vi "Select Channels and Update Properties.vi"(8 "error in (no error)":errorcluster, 11 "Node Ptr":u64) -> (0 "error out":errorcluster)   [LabVIEW 2015, in "J1939 Addon System Explorer.lvlib"]
uses:
  J1939 Addon System Explorer.lvlib
  <vilib>/NI VeriStand/Custom Device Tools/Custom Device Utility Library/Custom Device Utility Library.lvlib
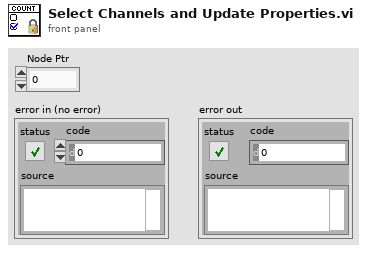
[diagram p1: front panel]
types:
  T1 = typedef "J1939 Addon System Explorer.lvlib/Protection Signal Settings.ctl" = cluster{"Input Channels":T2[], "Protection Type":T4}
  T2 = typedef "J1939 Addon System Explorer.lvlib/Protection Signal Linked Channels.ctl" = cluster{"Node Ref":T3}
  T3 = typedef "Custom Device API.lvlib/Custom Device Item Ref.ctl" = u64
  T4 = typedef "J1939 Addon Shared.lvlib/Protection Type.ctl" = enum16{"Arb ID + Bytes Checksum with Inversion", "Arb ID + Bytes CRC with Inversion", "Reversed Raw Signal Checksum with Inversion"}
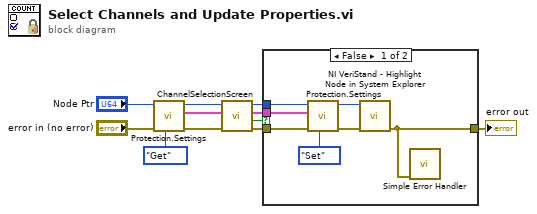
[diagram p0: block diagram]
diagram:
  n1 = call "Protection.Settings.vi"("Action"=enum8{"Get", "Set"}."Get", "error in"="error in (no error)", "Parent Ref"="Node Ptr") -> ("error out"=w3:errorcluster, "Selected Channels"=w10:T1, "Parent Ref Out"=w2:T3)  [unwired: 6 in]
  n2 = call "ChannelSelectionScreen.vi"("error in"=w3, "Selected Channels"=w10, "Parent Ref"=w2) -> ("error out"=w5:errorcluster, "Cancelled?"=w7:bool, "Selected Channels"=w11:T1, "Parent Ref Out"=w6:T3)  [unwired: 5 in]
  n3 = case shown="False" w7 {
    tunnel: w5 -> [w15 w19]
    tunnel: w6 -> [w13 _]
    tunnel: w11 -> [w14 _]
    tunnel: [w16 w19] -> w9
    frame False {
      n4 = call "Protection.Settings.vi"("Action"=enum8{"Get", "Set"}."Set", "error in"=w15, "Selected Channels"=w14, "Parent Ref"=w13) -> ("error out"=w17:errorcluster, "Parent Ref Out"=w18:T3)  [unwired: 5 in, 1 out]
      n5 = call <vilib>:"NI VeriStand - Highlight Node in System Explorer.vi"("error in (no error)"=w17, "Item Ref in"=w18) -> ("error out"=w16:errorcluster)  [unwired: 8 in, 1 out]
      n6 = call <vilib>:"Simple Error Handler.vi"("error in (no error)"=w16) -> ()  [unwired: 4 in, 5 out]
    }
    frame True {
    }
  }
  "error out" <- w9
